vi "bucle_medida_luz.vi"(8 "error in (no error)":errorcluster, 11 "msg":T1) -> (0 "error out":errorcluster, 3 "output cluster":T1={"mensaje"="", "info"={"I2C Slave Address "=0, "Data"=[0], "Bytes To Read"=0}, "LINX Resource"={"IO"=enum."Remote", "Interface"=enum."TCP", "LINX Device Config"={"Interface"=enum."TCP", "COM Port"="N/A", "TCP Configuration"={"IP Address"="panicattack", "Port"=6999}, "Device Family"=4, "Device ID"=1, "Device Name"="Raspberry Pi Model B", "TCP Ref"=refnum, "Channels"={"DI"=[2, 3, 4, 7, 8, 9, 10, 11, 14, 15, 17, 18, 22, 23, 24, 25, 27], "DO"=[2, 3, 4, 7, 8, 9, 10, 11, 14, 15, 17, 18, 22, 23, 24, 25, 27], "AI"=[], "AO"=[], "PWM"=[], "QE"=[], "UART"=[0], "I2C 2"=[0, 1], "SPI"=[0], "CAN"=[], "Servo"=[], "AI Ref (V)"=0.0, "AI Resolution (Bits)"=0, "AO Ref (V)"=0.0, "AO Resolution (Bits)"=0}}}})   [LabVIEW 2021]
uses:
  Ctls/msg.ctl
  <vilib>/MakerHub/LINX/Private/Type Defs/LINX Ref.ctl
  <vilib>/MakerHub/LINX/Private/Type Defs/Platform.ctl
  <vilib>/MakerHub/LINX/Private/Type Defs/Interface.ctl
  <vilib>/MakerHub/LINX/Private/Device/Type Defs/LINX Device Config.ctl
  <vilib>/MakerHub/LINX/Private/Device/Type Defs/TCP Config.ctl
  <vilib>/MakerHub/LINX/Private/Device/Type Defs/Channels.ctl
  <vilib>/MakerHub/LINX/LMH-LINX.lvlib
  <vilib>/MakerHub/LINX/Private/Device/Device.lvlib
panel:
  out "Data":u8[][](array[numeric])
  out "Datos Leídos":string[](array[string])
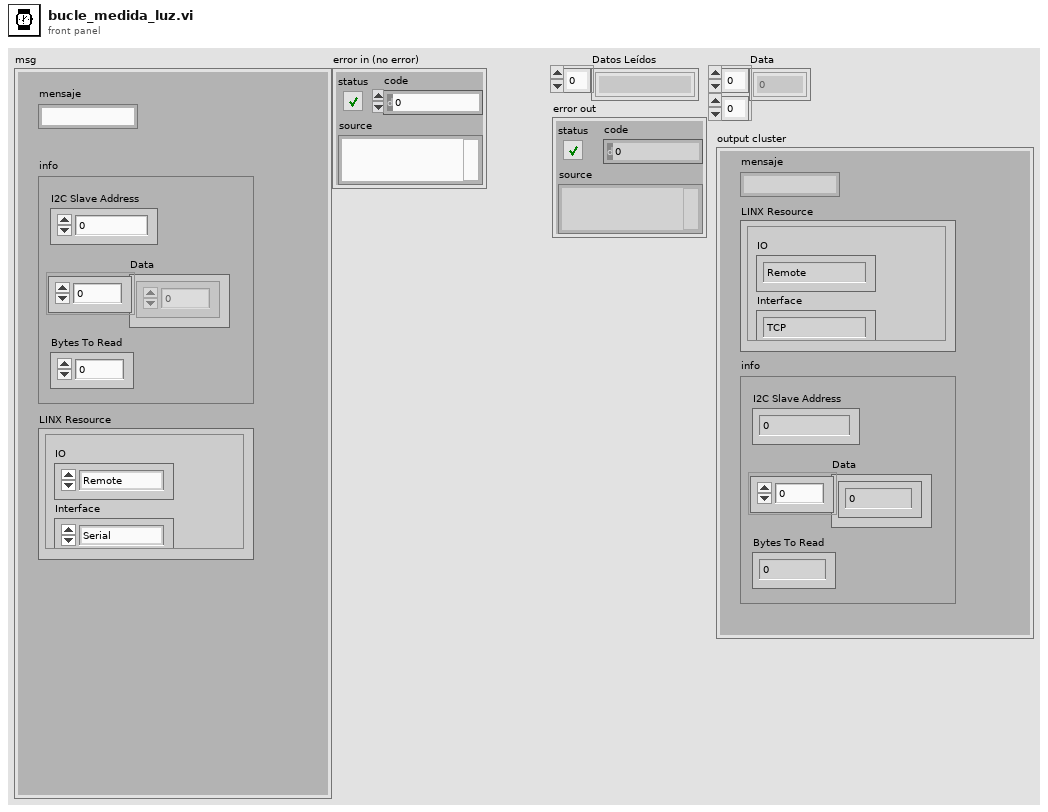
[diagram p1: front panel]
types:
  T1 = typedef "msg.ctl" = cluster{"mensaje":string, "info":cluster{"I2C Slave Address ":u8, "Data":u8[], "Bytes To Read":u8}, "LINX Resource":T2}
  T2 = typedef "LMH-LINX.lvlib/LINX Ref.ctl" = cluster{"IO":T3, "Interface":T4, "LINX Device Config":T5}
  T3 = typedef "LMH-LINX.lvlib/Platform.ctl" = enum16{"Remote", "Local"}
  T4 = typedef "LMH-LINX.lvlib/Interface.ctl" = enum16{"Serial", "TCP"}
  T5 = typedef "LMH-LINX.lvlib/Device.lvlib/LINX Device Config.ctl" = cluster{"Interface":T4, "COM Port":refnum<visa-resource-name>, "TCP Configuration":T6, "Device Family":u8, "Device ID":u8, "Device Name":string, "TCP Ref":refnum<k5>, "Channels":T7}
  T6 = typedef "LMH-LINX.lvlib/Device.lvlib/TCP Config.ctl" = cluster{"IP Address":string, "Port":u16}
  T7 = typedef "LMH-LINX.lvlib/Channels.ctl" = cluster{"DI":u8[], "DO":u8[], "AI":u8[], "AO":u8[], "PWM":u8[], "QE":u8[], "UART":u8[], "I2C 2":u8[], "SPI":u8[], "CAN":u8[], "Servo":u8[], "AI Ref (V)":dbl, "AI Resolution (Bits)":u8, "AO Ref (V)":dbl, "AO Resolution (Bits)":u8}
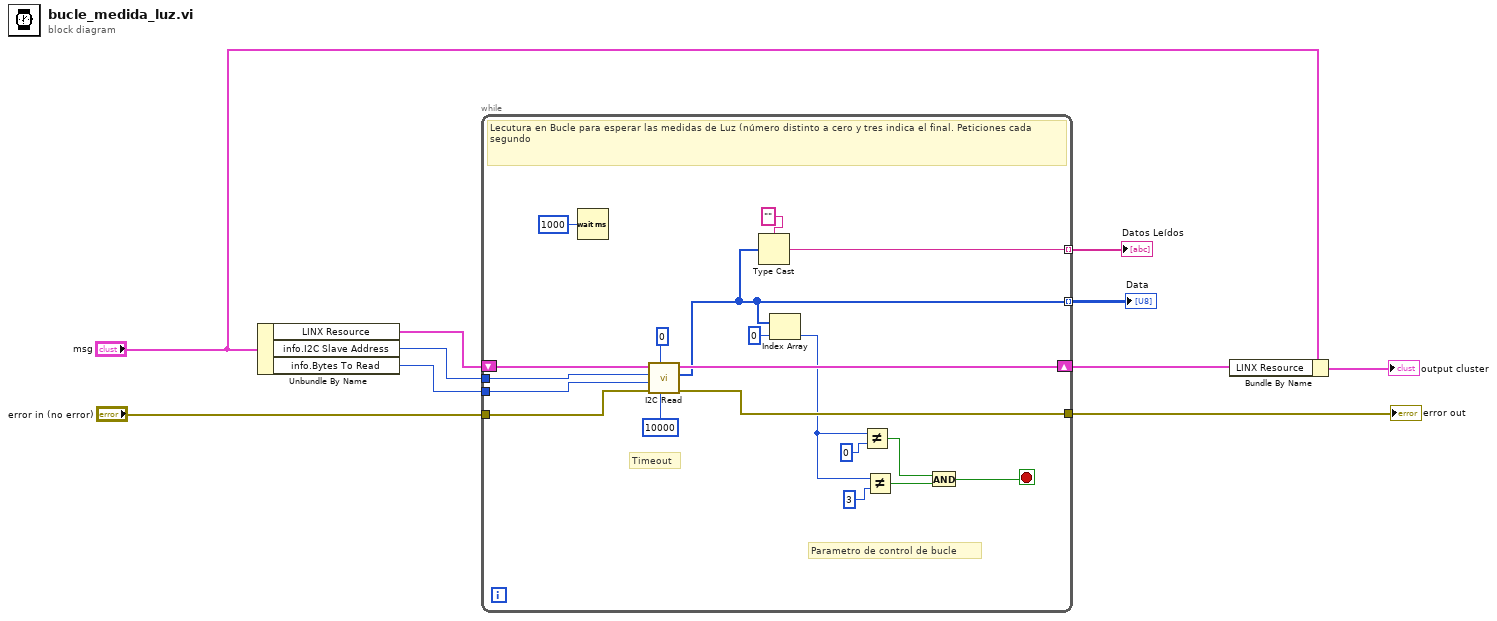
[diagram p0: block diagram]
diagram:
  n1 = Unbundle By Name("msg") -> ("LINX Resource"=w7:T2, "info.I2C Slave Address"=w9:u8, "info.Bytes To Read"=w10:u8)
  n2 = while {
    tunnel: w10 -> [w28]
    tunnel: w9 -> [w27]
    tunnel: "error in (no error)" -> [w25]
    shift-right: [w24] -> w2
    shift-left: w7 -> [w23]
    tunnel: [w19] -> w6 mode=indexing
    tunnel: [w18] -> w5
    tunnel: [w17] -> w4 mode=indexing
    stop <- w11 stop-if-true
    # "Parametro de control de bucle"
    # "Timeout"
    # "Lecutura en Bucle para esperar las medidas de Luz (número distinto a cero y tres indica el final. Peticiones cada segundo"
    n3 = Wait (ms)(milliseconds to wait=u32 1000) -> ()  [unwired: 1 out]
    n4 = call <vilib>:"I2C Read.vi"("Timeout (1000 ms)"=u16 10000, "I2C Channel"=u8 0, "Error In"=w25, "Bytes To Read"=w28, "I2C Slave Address (0)"=w27, "LINX Resource"=w23) -> ("Error Out"=w18:errorcluster, "Data"=w17:u8[], "LINX Resource"=w24:T2)  [unwired: 3 in]
    n5 = Type Cast(type="", x=w17) -> (*(type *) &x=w19:string)
    n6 = Index Array(array=w17, index=0) -> (element=w15:u8)
    n7 = Not Equal?(x=w15, y=u8 0) -> (x != y?=w13:bool)
    n8 = Not Equal?(x=w15, y=u8 3) -> (x != y?=w12:bool)
    n9 = And(x=w13, y=w12) -> (x .and. y?=w11:bool)
  }
  "Datos Leídos" <- w6
  "error out" <- w5
  "Data" <- w4
  n10 = Bundle By Name(cluster="msg", "LINX Resource"=w2) -> (→"output cluster":T1)
